vi "SERIAL_ResetDisplacementCommand.vi"(11 "navX Ref":T1={"SerialPortRef"={"DevStatus"={"status"=FALSE, "code"=0, "source"=""}, "Serial Port Name"=""}, "Board Information"={"WhoAmI (50 | 0x32)"=0, "Board Revision"=0, "Firmware Major Version"=0, "Firmware Minor Version"=0, "NAVX_BOARD_CAPABILITY"={"OMNIMOUNT"=FALSE, "YAW_RESET"=FALSE, "VEL_AND_DISP"=FALSE}, "NAVX_BOARD_YAW_AXIS"={"BOARD_YAW_AXIS_UP"=FALSE, "BOARD_YAW_AXIS"=0}}, "Status"={"Update Rate Hz"=0, "Accelerometer Full-Scale Range"=0, "Gyro Full-Scale Range"=0, "NAVX_OP_STATUS"=0, "NAVX_CAL_STATUS"=0, "NAVX_SELFTEST_STATUS"=0, "NAVX_SENSOR_STATUS"={"MOVING"=FALSE, "YAW_STABLE"=FALSE, "MAG_DISTURBANCE"=FALSE, "ALTITUDE_VALID"=FALSE, "SEALEVEL_PRESS_SET"=FALSE, "FUSED_HEADING_VALID"=FALSE}}, "Offsets"={"Yaw"=0.0, "Quat W"=0.0, "Quat X"=0.0, "Quat Y"=0.0, "Quat Z"=0.0}, "Update Rate (4Hz-60Hz)"=50, "Nav6Mode (YPR)"=enum."YPR", "refnum name"="", "error"={"status"=FALSE, "code"=0, "source"=""}, "Loop VI Refnum"=refnum, "Serial Port"=enum."Onboard RS-232"} {"Status"."NAVX_OP_STATUS" items=["INITIALIZING", "SELFTEST_IN_PROGRESS", "ERROR", "IMU_AUTOCAL_IN_PROGRESS", "NORMAL"]; "Status"."NAVX_CAL_STATUS" items=["IMU_CAL_STATE_MASK"=3, "IMU_CAL_INPROGRESS"=0, "IMU_CAL_ACCUMULATE"=1, "IMU_CAL_COMPLETE"=2, "MAG_CAL_COMPLETE"=4, "BARO_CAL_COMPLETE"=8]}) -> (3 "navX Ref":T1={"SerialPortRef"={"DevStatus"={"status"=FALSE, "code"=0, "source"=""}, "Serial Port Name"=""}, "Board Information"={"WhoAmI (50 | 0x32)"=0, "Board Revision"=0, "Firmware Major Version"=0, "Firmware Minor Version"=0, "NAVX_BOARD_CAPABILITY"={"OMNIMOUNT"=FALSE, "YAW_RESET"=FALSE, "VEL_AND_DISP"=FALSE}, "NAVX_BOARD_YAW_AXIS"={"BOARD_YAW_AXIS_UP"=FALSE, "BOARD_YAW_AXIS"=0}}, "Status"={"Update Rate Hz"=0, "Accelerometer Full-Scale Range"=0, "Gyro Full-Scale Range"=0, "NAVX_OP_STATUS"=0, "NAVX_CAL_STATUS"=0, "NAVX_SELFTEST_STATUS"=0, "NAVX_SENSOR_STATUS"={"MOVING"=FALSE, "YAW_STABLE"=FALSE, "MAG_DISTURBANCE"=FALSE, "ALTITUDE_VALID"=FALSE, "SEALEVEL_PRESS_SET"=FALSE, "FUSED_HEADING_VALID"=FALSE}}, "Offsets"={"Yaw"=0.0, "Quat W"=0.0, "Quat X"=0.0, "Quat Y"=0.0, "Quat Z"=0.0}, "Update Rate (4Hz-60Hz)"=50, "Nav6Mode (YPR)"=enum."YPR", "refnum name"="", "error"={"status"=FALSE, "code"=0, "source"=""}, "Loop VI Refnum"=refnum, "Serial Port"=enum."Onboard RS-232"} {"Status"."NAVX_OP_STATUS" items=["INITIALIZING", "SELFTEST_IN_PROGRESS", "ERROR", "IMU_AUTOCAL_IN_PROGRESS", "NORMAL"]; "Status"."NAVX_CAL_STATUS" items=["IMU_CAL_STATE_MASK"=3, "IMU_CAL_INPROGRESS"=0, "IMU_CAL_ACCUMULATE"=1, "IMU_CAL_COMPLETE"=2, "MAG_CAL_COMPLETE"=4, "BARO_CAL_COMPLETE"=8]})   [LabVIEW 2014, in "navX-MXP IMU.lvlib"]
uses:
  navX-MXP IMU.lvlib
  navX Serial DevRef.ctl
  <vilib>/Rock Robotics/WPI/SerialPort/WPI_SerialPortRef.ctl
  COMMON/TypeDefs/Data TypeDefs/navX Board Information.ctl
  COMMON/TypeDefs/Value TypeDefs/navX NAVX_BOARD_CAPABILITY.ctl
  COMMON/TypeDefs/Value TypeDefs/navX NAVX_BOARD_YAW_AXIS.ctl
  COMMON/TypeDefs/Data TypeDefs/navX Status Data.ctl
  COMMON/TypeDefs/Value TypeDefs/navX NAVX_OP_STATUS.ctl
  COMMON/TypeDefs/Value TypeDefs/navX NAVX_CAL_STATUS.ctl
  COMMON/TypeDefs/Value TypeDefs/navX NAVX_SENSOR_STATUS.ctl
  TypeDefs/navX Serial Mode.ctl
  IO/NI WPI/WPI_SerialPort_USB.ctl
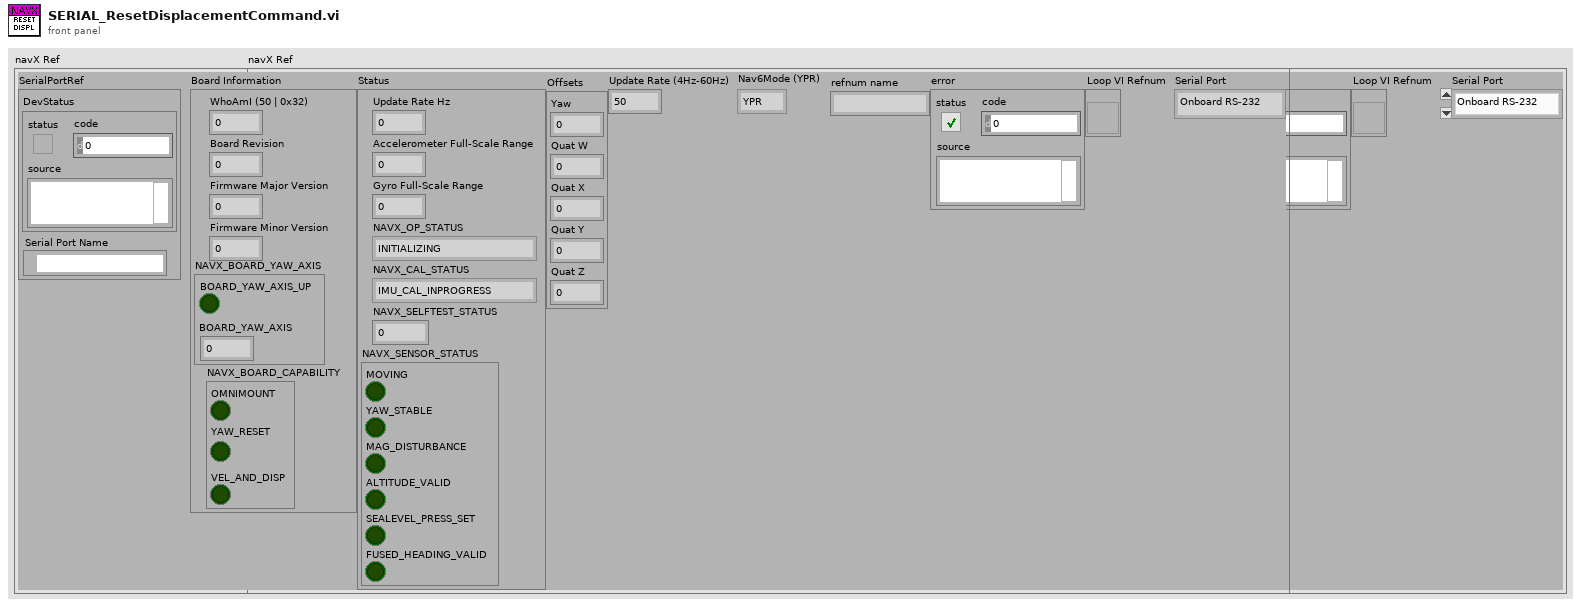
[diagram p1: front panel]
types:
  T1 = typedef "navX-MXP IMU.lvlib/navX Serial DevRef.ctl" = cluster{"SerialPortRef":T2, "Board Information":T3, "Status":T6, "Offsets":cluster{"Yaw":dbl, "Quat W":dbl, "Quat X":dbl, "Quat Y":dbl, "Quat Z":dbl}, "Update Rate (4Hz-60Hz)":u8, "Nav6Mode (YPR)":T10, "refnum name":string, "error":errorcluster, "Loop VI Refnum":refnum<vi>, "Serial Port":T11}
  T2 = typedef "WPI_SerialPortRef.ctl" = cluster{"DevStatus":errorcluster, "Serial Port Name":refnum<visa-resource-name>}
  T3 = typedef "navX-MXP IMU.lvlib/navX Board Information.ctl" = cluster{"WhoAmI (50 | 0x32)":u8, "Board Revision":u8, "Firmware Major Version":u8, "Firmware Minor Version":u8, "NAVX_BOARD_CAPABILITY":T4, "NAVX_BOARD_YAW_AXIS":T5}
  T4 = typedef "navX-MXP IMU.lvlib/navX NAVX_BOARD_CAPABILITY.ctl" = cluster{"OMNIMOUNT":bool, "YAW_RESET":bool, "VEL_AND_DISP":bool}
  T5 = typedef "navX-MXP IMU.lvlib/navX NAVX_BOARD_YAW_AXIS.ctl" = cluster{"BOARD_YAW_AXIS_UP":bool, "BOARD_YAW_AXIS":u8}
  T6 = typedef "navX-MXP IMU.lvlib/navX Status Data.ctl" = cluster{"Update Rate Hz":u8, "Accelerometer Full-Scale Range":u8, "Gyro Full-Scale Range":u16, "NAVX_OP_STATUS":T7, "NAVX_CAL_STATUS":T8, "NAVX_SELFTEST_STATUS":u8, "NAVX_SENSOR_STATUS":T9}
  T7 = typedef "navX-MXP IMU.lvlib/navX NAVX_OP_STATUS.ctl" = u8
  T8 = typedef "navX-MXP IMU.lvlib/navX NAVX_CAL_STATUS.ctl" = u8
  T9 = typedef "navX-MXP IMU.lvlib/navX NAVX_SENSOR_STATUS.ctl" = cluster{"MOVING":bool, "YAW_STABLE":bool, "MAG_DISTURBANCE":bool, "ALTITUDE_VALID":bool, "SEALEVEL_PRESS_SET":bool, "FUSED_HEADING_VALID":bool}
  T10 = typedef "navX-MXP IMU.lvlib/navX Serial Mode.ctl" = enum16{"YPR", "Gyro", "Quaternion", "AHRS", "AHRSPos"}
  T11 = typedef "navX-MXP IMU.lvlib/WPI_SerialPort_USB.ctl" = enum16{"Onboard RS-232", "MXP TTL", "USB"}
  T12 = typedef "navX-MXP IMU.lvlib/navX YPRH Data.ctl" = cluster{"Yaw":dbl, "Pitch":dbl, "Roll":dbl, "Heading":dbl}
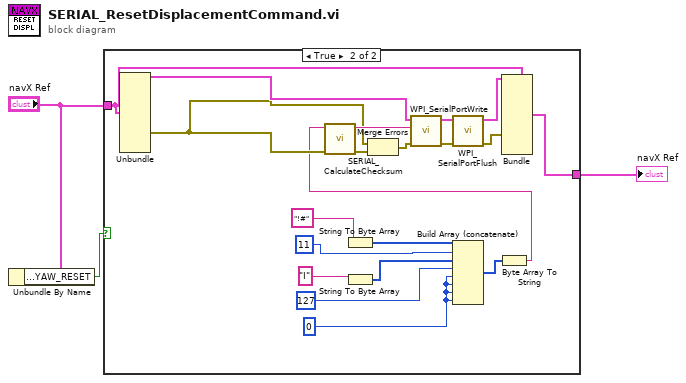
[diagram p0: block diagram]
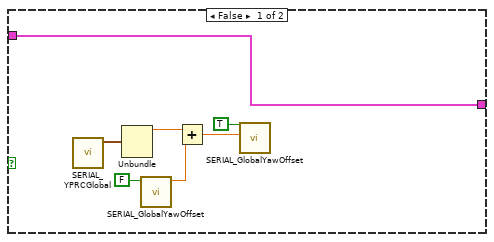
[diagram p2: hidden frame]
diagram:
  n1 = Unbundle By Name("navX Ref") -> ("Board Information.NAVX_BOARD_CAPABILITY.YAW_RESET"=w1:bool)
  n2 = case shown="True" w1 {
    tunnel: [w9 w27] -> w3
    tunnel: "navX Ref" -> [w9 w13]
    frame False {
      n3 = call "SERIAL_YPRCGlobal.vi"() -> ("YPRH"=w10:T12)  [unwired: 10 in, 1 out]
      n4 = Unbundle(w10) -> ("Yaw"=w5:dbl)  [unwired: 3 out]
      n5 = call "SERIAL_GlobalYawOffset.vi"("Set"=FALSE) -> ("OutputYawOffset"=w6:dbl)  [unwired: 10 in]
      n6 = Add(x=w5, y=w6) -> (x+y=w4:dbl)
      n7 = call "SERIAL_GlobalYawOffset.vi"("InputYawOffset"=w4, "Set"=TRUE) -> ()  [unwired: 9 in, 1 out]
    }
    frame True {
      w12 = u8 0 ("lower limit")
      n8 = Unbundle(w13) -> ("SerialPortRef"=w22:T2, "error"=w18:errorcluster)  [unwired: 8 out]
      n9 = String To Byte Array(string="!#" ("format string")) -> (unsigned byte array=w20:u8[])
      n10 = String To Byte Array(string="I" ("format string")) -> (unsigned byte array=w11:u8[])
      n11 = Build Array (concatenate)(w20, u8 11 ("lower limit"), w11, u8 127 ("lower limit"), w12, w12, w12, w12) -> (w19:u8[])
      n12 = Byte Array To String(unsigned byte array=w19) -> (string=w17:string)
      n13 = call "SERIAL_CalculateChecksum.vi"("error in"=w18, "Content"=w17) -> ("error out"=w24:errorcluster, "Teminated Content"=w26:string)  [unwired: 4 in]
      n14 = Merge Errors(w18, w24) -> (w25:errorcluster)
      n15 = call <vilib>:"WPI_SerialPortWrite.vi"("error in (no error)"=w25, "Buffer"=w26, "SerialPortRef"=w22) -> ("error out"=w30:errorcluster, "SerialPortRef"=w29:T2)  [unwired: 6 in, 1 out]
      n16 = call <vilib>:"WPI_SerialPortFlush.vi"("error in (no error)"=w30, "SerialPortRef"=w29) -> ("error out"=w23:errorcluster, "SerialPortRef"=w28:T2)  [unwired: 8 in]
      n17 = Bundle(cluster=w13, "SerialPortRef"=w28, "error"=w23) -> (w27:T1)  [unwired: 8 in]
    }
  }
  "navX Ref" <- w3
